vi "fgv_reg_ref.vi"(7 "cmd":T2, 11 "output cluster":T1) -> (3 "output cluster 2":T1)   [LabVIEW 2019]
uses:
  _ctrl/rw.ctl
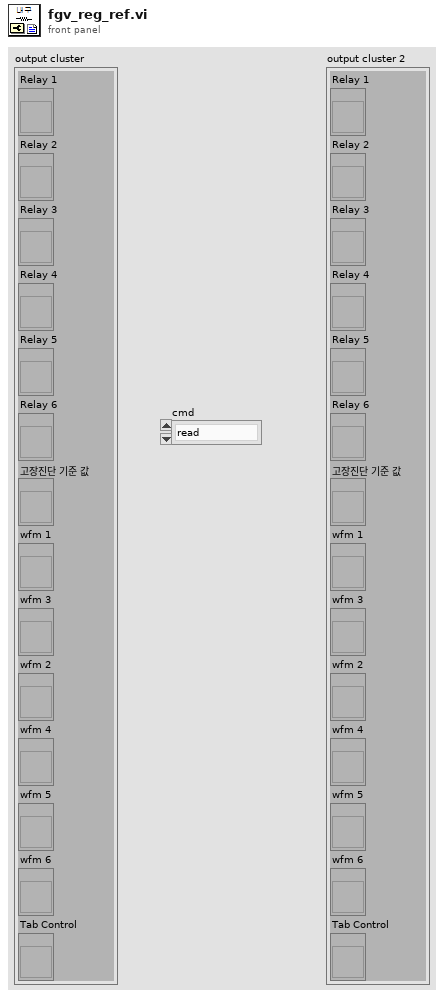
[diagram p1: front panel]
types:
  T1 = cluster{"Relay 1":refnum<vi>, "Relay 2":refnum<vi>, "Relay 3":refnum<vi>, "Relay 4":refnum<vi>, "Relay 5":refnum<vi>, "Relay 6":refnum<vi>, "고장진단 기준 값":refnum<vi>, "wfm 1":refnum<vi>, "wfm 3":refnum<vi>, "wfm 2":refnum<vi>, "wfm 4":refnum<vi>, "wfm 5":refnum<vi>, "wfm 6":refnum<vi>, "Tab Control":refnum<vi>}
  T2 = typedef "rw.ctl" = enum16{"read", "write"}
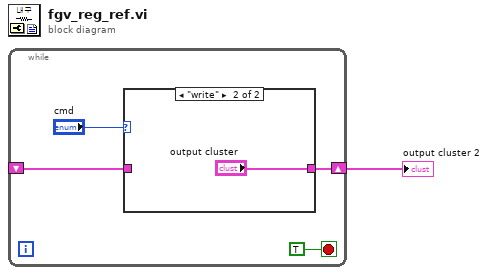
[diagram p0: block diagram]
diagram:
  n1 = while {
    shift-right: [w3] -> w1
    shift-left: _ -> [w2]
    stop <- TRUE stop-if-true
    n2 = case shown="\"write\"" "cmd" {
      tunnel: [w6 "output cluster"] -> w3
      tunnel: w2 -> [w6 _]
      frame "read", Default {
      }
      frame "write" {
      }
    }
  }
  "output cluster 2" <- w1
